vi "Camera_Change Settings.vi"(8 "Error":errorcluster, 9 "Camera Settings":T1 {"Saturation" min=0 max=100 step=1; "Sharpness" min=0 max=100 step=1; "Brightness" min=0 max=100 step=1; "Exposure (%)" min=0.0 max=100.0 step=1.0}, 11 "CameraDevRef":T6) -> (0 "Error Out":errorcluster, 3 "CameraDevRef Out":T6)   [LabVIEW 2017, in "VisionSystem.lvlib"]
uses:
  VisionSystem.lvlib
  <vilib>/Rock Robotics/WPI/Camera/WPI_CameraDevRef.ctl
  TypeDefs/Cluster_Camera Settings.ctl
  <vilib>/Rock Robotics/WPI/Camera/WPI_CameraImageSize.ctl
  <vilib>/Rock Robotics/WPI/Camera/WPI_CameraFrameRate.ctl
  <vilib>/Rock Robotics/WPI/Camera/WPI_CameraWhite Balance Values.ctl
  <vilib>/Rock Robotics/WPI/Camera/WPI_CameraExposure Values.ctl
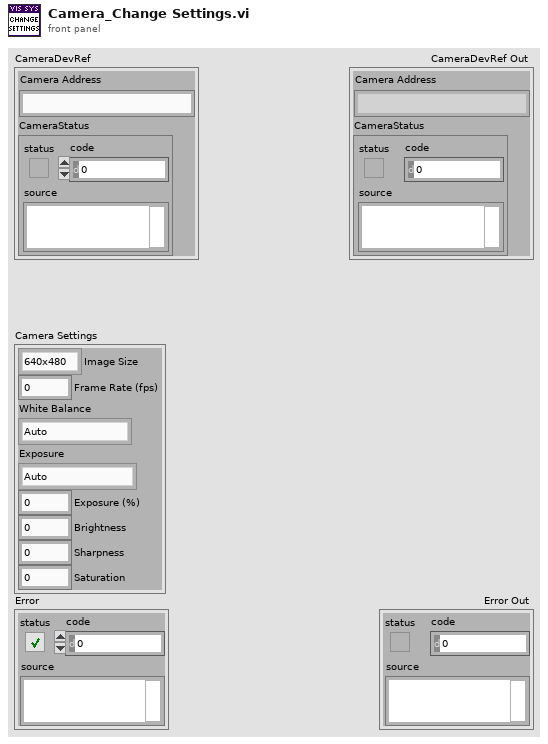
[diagram p1: front panel]
types:
  T1 = typedef "Cluster_Camera Settings.ctl" = cluster{"Image Size":T2, "Frame Rate (fps)":T3, "White Balance":T4, "Exposure":T5, "Exposure (%)":dbl, "Brightness":i32, "Sharpness":i32, "Saturation":i32}
  T2 = typedef "WPI_CameraImageSize.ctl" = enum16{"640x480", "320x240", "160x120", "Custom"}
  T3 = typedef "WPI_CameraFrameRate.ctl" = u32
  T4 = typedef "WPI_CameraWhite Balance Values.ctl" = enum16{"Auto", "Fixed indoor", "Fixed outdoor 1", "Fixed outdoor 2", "Fixed fluorescent 1", "Fixed fluorescent 2", "Hold current", "Custom"}
  T5 = typedef "WPI_CameraExposure Values.ctl" = enum16{"Auto", "Flicker-free 50 Hz", "Flicker-free 60 Hz", "Hold current", "Custom"}
  T6 = typedef "WPI_CameraDevRef.ctl" = cluster{"Camera Address":string, "CameraStatus":errorcluster}
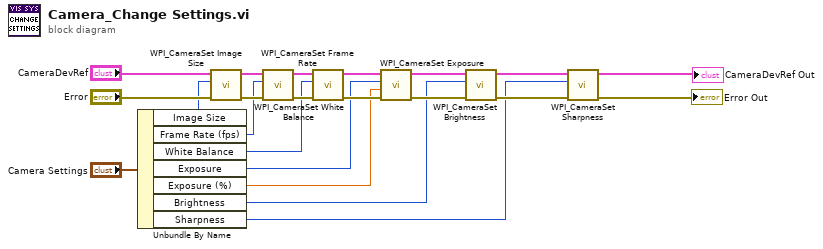
[diagram p0: block diagram]
diagram:
  n1 = Unbundle By Name("Camera Settings") -> ("Image Size"=w13:T2, "Frame Rate (fps)"=w12:T3, "White Balance"=w11:T4, "Exposure"=w10:T5, "Exposure (%)"=w9:dbl, "Brightness"=w2:i32, "Sharpness"=w1:i32)
  n2 = call <vilib>:"WPI_CameraSet Image Size.vi"("error in (no error)"="Error", "Image Size"=w13, "CameraDevRef"="CameraDevRef") -> ("error out"=w17:errorcluster, "CameraDevRef Out"=w20:T6)  [unwired: 1 in, 6 out]
  n3 = call <vilib>:"WPI_CameraSet Frame Rate.vi"("error in (no error)"=w17, "Frame Rate (fps)"=w12, "CameraDevRef"=w20) -> ("error out"=w16:errorcluster, "CameraDevRef Out"=w22:T6)  [unwired: 7 out]
  n4 = call <vilib>:"WPI_CameraSet White Balance.vi"("error in (no error)"=w16, "White Balance"=w11, "CameraDevRef"=w22) -> ("error out"=w15:errorcluster, "CameraDevRef Out"=w21:T6)  [unwired: 1 in, 6 out]
  n5 = call <vilib>:"WPI_CameraSet Exposure.vi"("error in (no error)"=w15, "Exposure (%)"=w9, "Exposure"=w10, "CameraDevRef"=w21) -> ("error out"=w3:errorcluster, "CameraDevRef Out"=w4:T6)  [unwired: 6 out]
  n6 = call <vilib>:"WPI_CameraSet Brightness.vi"("error in (no error)"=w3, "Brightness"=w2, "CameraDevRef"=w4) -> ("error out"=w6:errorcluster, "CameraDevRef Out"=w8:T6)  [unwired: 1 in, 6 out]
  n7 = call <vilib>:"WPI_CameraSet Sharpness.vi"("error in (no error)"=w6, "Sharpness"=w1, "CameraDevRef"=w8) -> ("error out"=→"Error Out":errorcluster, "CameraDevRef Out"=→"CameraDevRef Out":T6)  [unwired: 7 in]
